vi "MGCC_EnergyMgmt_EMS_HTB_test.vi"() -> ()   [LabVIEW 2016]
uses:
  <vilib>/imath/engines/lvmath2/RunTimeEngine/NodeEndStatement/NIMS_NodeEndStatement_Output.vi
  <instcachedir>/0/NIMS_NodeEndStatement_Output_53EC0D466D134D7ABD903AC30B43404B.lvgen/NIMS_NodeEndStatement_Output_53EC0D466D134D7ABD903AC30B43404B_005.vi
  <instcachedir>/0/NIMS_NodeEndStatement_Output_53EC0D466D134D7ABD903AC30B43404B.lvgen/NIMS_NodeEndStatement_Output_53EC0D466D134D7ABD903AC30B43404B_001.vi
  <vilib>/imath/engines/lvmath2/RunTimeEngine/ErrorHandling/NIMS_Finalize Error.vi
  <vilib>/imath/engines/lvmath2/RunTimeEngine/BuiltInFunctions/is_nan/NIMS_is_nan.vi
  <instcachedir>/0/NIMS_is_nan_BCCD798162CC49E3A8E57072444F6EB6.lvgen/NIMS_is_nan_BCCD798162CC49E3A8E57072444F6EB6_003.vi
  <vilib>/imath/engines/lvmath2/RunTimeEngine/BuiltInFunctions/sum/NIMS_sum(GV).vi
  <instcachedir>/0/NIMS_sum(GV)_67F5EC36BC034E54A6BEC5B0673C00E5.lvgen/NIMS_sum(GV)_67F5EC36BC034E54A6BEC5B0673C00E5_000.vi
  <vilib>/imath/engines/lvmath2/RunTimeEngine/BuiltInFunctions/max/1 input/NIMS_max(RV).vi
  <instcachedir>/0/NIMS_max(RV)_237633DB1D604D5BA7001287DF3C7957.lvgen/NIMS_max(RV)_237633DB1D604D5BA7001287DF3C7957_002.vi
  <vilib>/imath/engines/lvmath2/RunTimeEngine/MatrixToken/NIMS_MatrixToken_RV_RV.vi
  <instcachedir>/0/NIMS_MatrixToken_RV_RV_41289AEE7DB340EFBB9CA44FA48DA89B.lvgen/NIMS_MatrixToken_RV_RV_41289AEE7DB340EFBB9CA44FA48DA89B_002.vi
  <vilib>/imath/engines/lvmath2/RunTimeEngine/MatrixToken/NIMS_MatrixToken_M_SorCV.vi
  <instcachedir>/0/NIMS_MatrixToken_M_SorCV_D3266533510A4291A747E91CF193467A.lvgen/NIMS_MatrixToken_M_SorCV_D3266533510A4291A747E91CF193467A_000.vi
  <vilib>/imath/engines/lvmath2/RunTimeEngine/ErrorHandling/NIMS_Create Error From Enums.vi
  <vilib>/imath/engines/lvmath2/RunTimeEngine/BuiltInFunctions/tril/NIMS_tril.vi
  <instcachedir>/0/NIMS_tril_6D22CCA5CB604C1FB8874D0E0A590B2C.lvgen/NIMS_tril_6D22CCA5CB604C1FB8874D0E0A590B2C_003.vi
  <vilib>/imath/engines/lvmath2/RunTimeEngine/RowToken/NIMS_RowToken_M_M.vi
  <instcachedir>/0/NIMS_RowToken_M_M_968CDE3545E74ACDAEA4B48DE01EEECA.lvgen/NIMS_RowToken_M_M_968CDE3545E74ACDAEA4B48DE01EEECA_005.vi
  <vilib>/imath/engines/lvmath2/RunTimeEngine/RowToken/NIMS_RowToken_M_CV.vi
  <instcachedir>/0/NIMS_RowToken_M_CV_FA79F1D1D17D44459F3ED8E09EE8B625.lvgen/NIMS_RowToken_M_CV_FA79F1D1D17D44459F3ED8E09EE8B625_002.vi
  <vilib>/imath/engines/lvmath2/RunTimeEngine/MatrixToken/NIMS_MatrixToken_M_M.vi
  <instcachedir>/0/NIMS_MatrixToken_M_M_DF273B0CC20F424BBF1EDA9F4E71C841.lvgen/NIMS_MatrixToken_M_M_DF273B0CC20F424BBF1EDA9F4E71C841_005.vi
  <vilib>/imath/engines/lvmath2/RunTimeEngine/ArithmeticOperatorToken/NIMS_ArithmeticOperator_minus.vi
  <instcachedir>/0/NIMS_ArithmeticOperator_minus_E3B65B1D26A44BB184AFDC5B3F458E3D.lvgen/NIMS_ArithmeticOperator_minus_E3B65B1D26A44BB184AFDC5B3F458E3D_003.vi
  <vilib>/imathl/engines/lvmath/Functions/Error Handling/Create Error.vi
  <vilib>/imath/engines/lvmath2/RunTimeEngine/BuiltInFunctions/double/NIMS_double.vi
  <instcachedir>/0/NIMS_double_34E32F64C2B04A25A042F4CA881A0A41.lvgen/NIMS_double_34E32F64C2B04A25A042F4CA881A0A41_000.vi
  <instcachedir>/0/NIMS_double_34E32F64C2B04A25A042F4CA881A0A41.lvgen/NIMS_double_34E32F64C2B04A25A042F4CA881A0A41_002.vi
  <vilib>/imath/engines/lvmath2/RunTimeEngine/BuiltInFunctions/length/NIMS_length(GV).vi
  <instcachedir>/0/NIMS_length(GV)_08A3D13377FD4E4B96F5795FBF3698FA.lvgen/NIMS_length(GV)_08A3D13377FD4E4B96F5795FBF3698FA_000.vi
  <vilib>/imath/engines/lvmath2/RunTimeEngine/BuiltInFunctions/zeros/NIMS_V=zeros(I32,I32).vi
  <vilib>/imath/engines/lvmath2/RunTimeEngine/BuiltInFunctions/ones/NIMS_V=ones(I32,I32).vi
  <vilib>/imath/engines/lvmath2/RunTimeEngine/RangeToken/NIMS_Range_R2 - Integer.vi
  <instcachedir>/0/NIMS_Range_R2 - Integer_89B873E74E6E489885E44F751DD9C6BF.lvgen/NIMS_Range_R2 - Integer_89B873E74E6E489885E44F751DD9C6BF_000.vi
  <vilib>/imath/engines/lvmath2/RunTimeEngine/CommandStatement/MC_CommandStatement_break.vi
  <vilib>/imath/engines/lvmath2/RunTimeEngine/IndexRead/NIMS V(S).vi
  <instcachedir>/0/NIMS V(S)_0488751826AF41519A22953C041130DC.lvgen/NIMS V(S)_0488751826AF41519A22953C041130DC_000.vi
  <vilib>/imath/engines/lvmath2/RunTimeEngine/BuiltInFunctions/is_inf/NIMS_is_inf.vi
  <instcachedir>/0/NIMS_is_inf_B756F33AF9174A0299BAA1DAC25DCC60.lvgen/NIMS_is_inf_B756F33AF9174A0299BAA1DAC25DCC60_002.vi
  <vilib>/imath/engines/lvmath2/RunTimeEngine/IndexReplace/NIMS V(S)=S.vi
  <instcachedir>/0/NIMS V(S)=S_57E16554CB8B4B90AAB163894F717546.lvgen/NIMS V(S)=S_57E16554CB8B4B90AAB163894F717546_003.vi
  <instcachedir>/0/NIMS_MatrixToken_M_M_DF273B0CC20F424BBF1EDA9F4E71C841.lvgen/NIMS_MatrixToken_M_M_DF273B0CC20F424BBF1EDA9F4E71C841_004.vi
  <vilib>/imath/engines/lvmath2/RunTimeEngine/BuiltInFunctions/findnz/NIMS_[3o]_findnz(GM).vi
  <instcachedir>/0/NIMS_[3o]_findnz(GM)_99A5867F30DB48758370F82C3149E97C.lvgen/NIMS_[3o]_findnz(GM)_99A5867F30DB48758370F82C3149E97C_003.vi
  <vilib>/imath/engines/lvmath2/RunTimeEngine/MatrixToken/NIMS_MatrixToken_SorCV_M.vi
  <instcachedir>/0/NIMS_MatrixToken_SorCV_M_667D6DA9EAAA4E73AD685CBB2779BCDB.lvgen/NIMS_MatrixToken_SorCV_M_667D6DA9EAAA4E73AD685CBB2779BCDB_000.vi
  <instcachedir>/0/NIMS_NodeEndStatement_Output_53EC0D466D134D7ABD903AC30B43404B.lvgen/NIMS_NodeEndStatement_Output_53EC0D466D134D7ABD903AC30B43404B_004.vi
  <instcachedir>/0/NIMS_NodeEndStatement_Output_53EC0D466D134D7ABD903AC30B43404B.lvgen/NIMS_NodeEndStatement_Output_53EC0D466D134D7ABD903AC30B43404B_010.vi
  <vilib>/imath/engines/lvmath2/RunTimeEngine/IndexRead/NIMS V(R2).vi
  <instcachedir>/0/NIMS V(R2)_C76619605A0E4E9F8B2FA9389712AC47.lvgen/NIMS V(R2)_C76619605A0E4E9F8B2FA9389712AC47_000.vi
  <instcachedir>/0/NIMS_max(RV)_237633DB1D604D5BA7001287DF3C7957.lvgen/NIMS_max(RV)_237633DB1D604D5BA7001287DF3C7957_000.vi
  <vilib>/imath/engines/lvmath2/RunTimeEngine/ArithmeticOperatorToken/NIMS_ArithmeticOperator_times.vi
  <instcachedir>/0/NIMS_ArithmeticOperator_times_953B34F74CAC448FB707D816A29CC5F0.lvgen/NIMS_ArithmeticOperator_times_953B34F74CAC448FB707D816A29CC5F0_000.vi
  liblp_solver.so
panel:
  out "Net load after":dbl[](graph)
  out "Net load b4":dbl[](graph)
  out "Battery2 Dispatch":dbl[](graph)
  out "Battery1 Dispatch":dbl[](graph)
  out "Savings":dbl
  out "return type":i32
  out "error out":errorcluster
  out "Forecast PV":dbl[](graph)
  out "Forecast Load":dbl[](graph)
  out "err_flg":i32
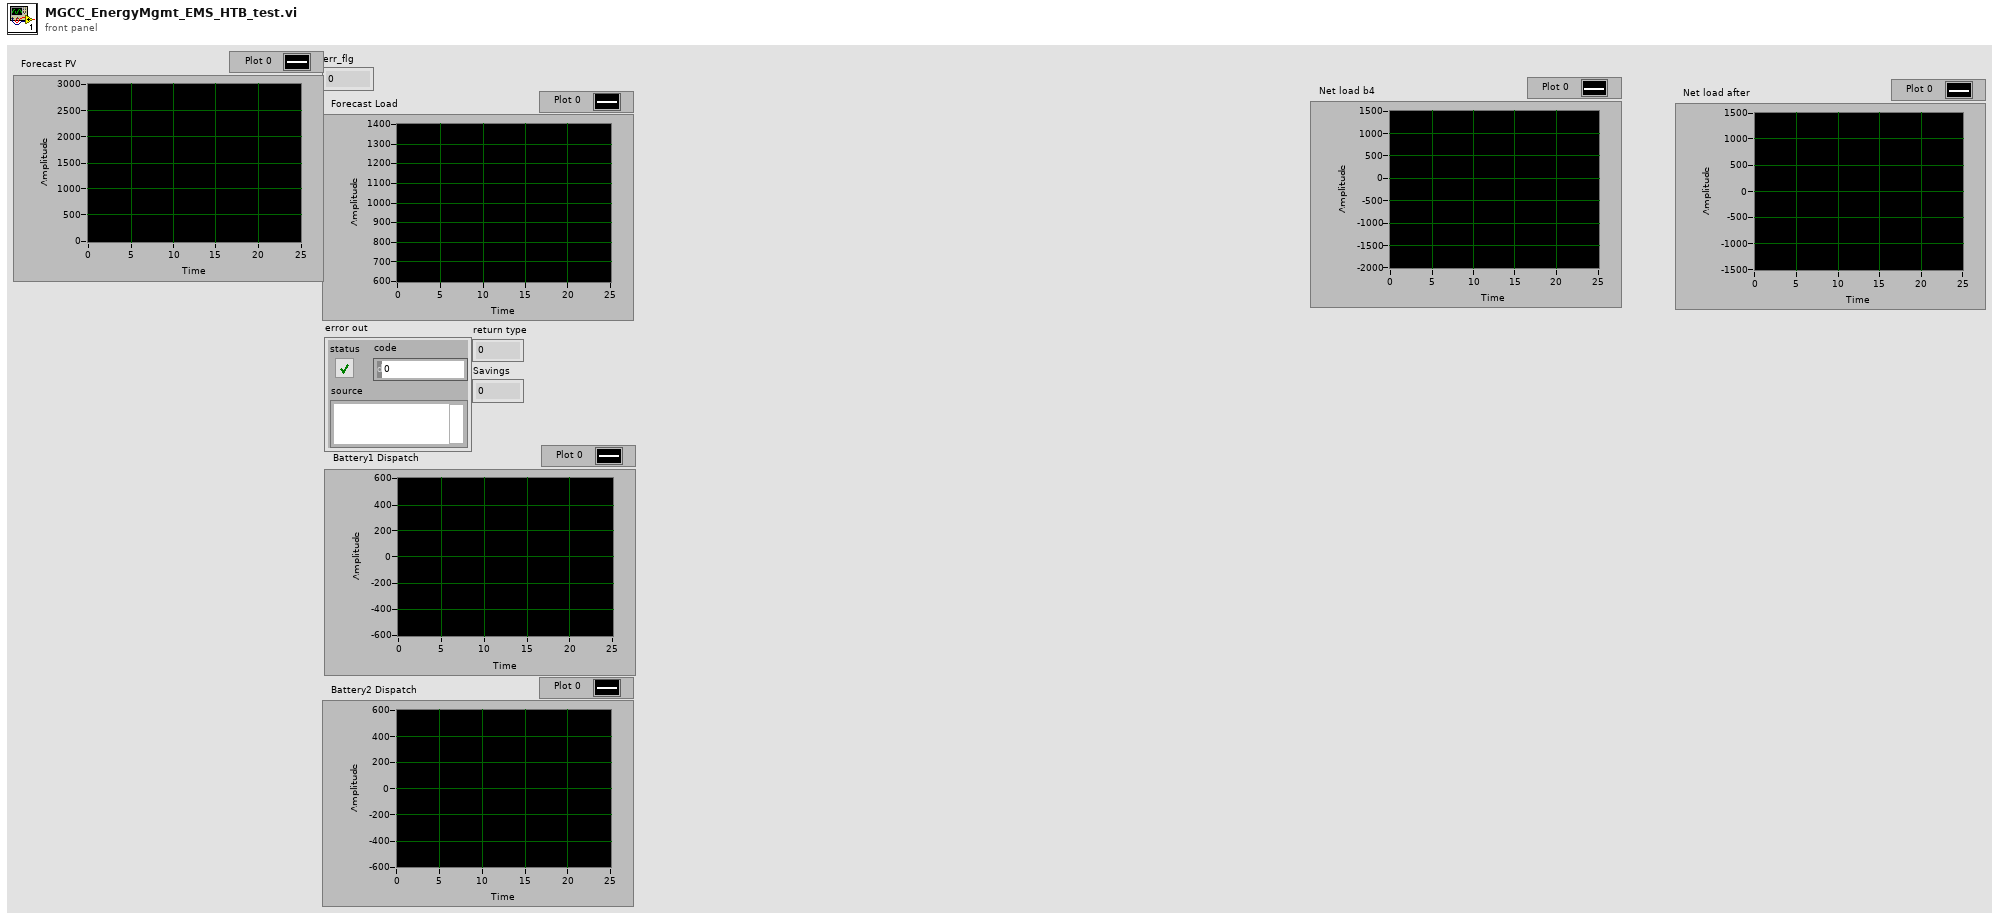
[diagram p1: front panel]
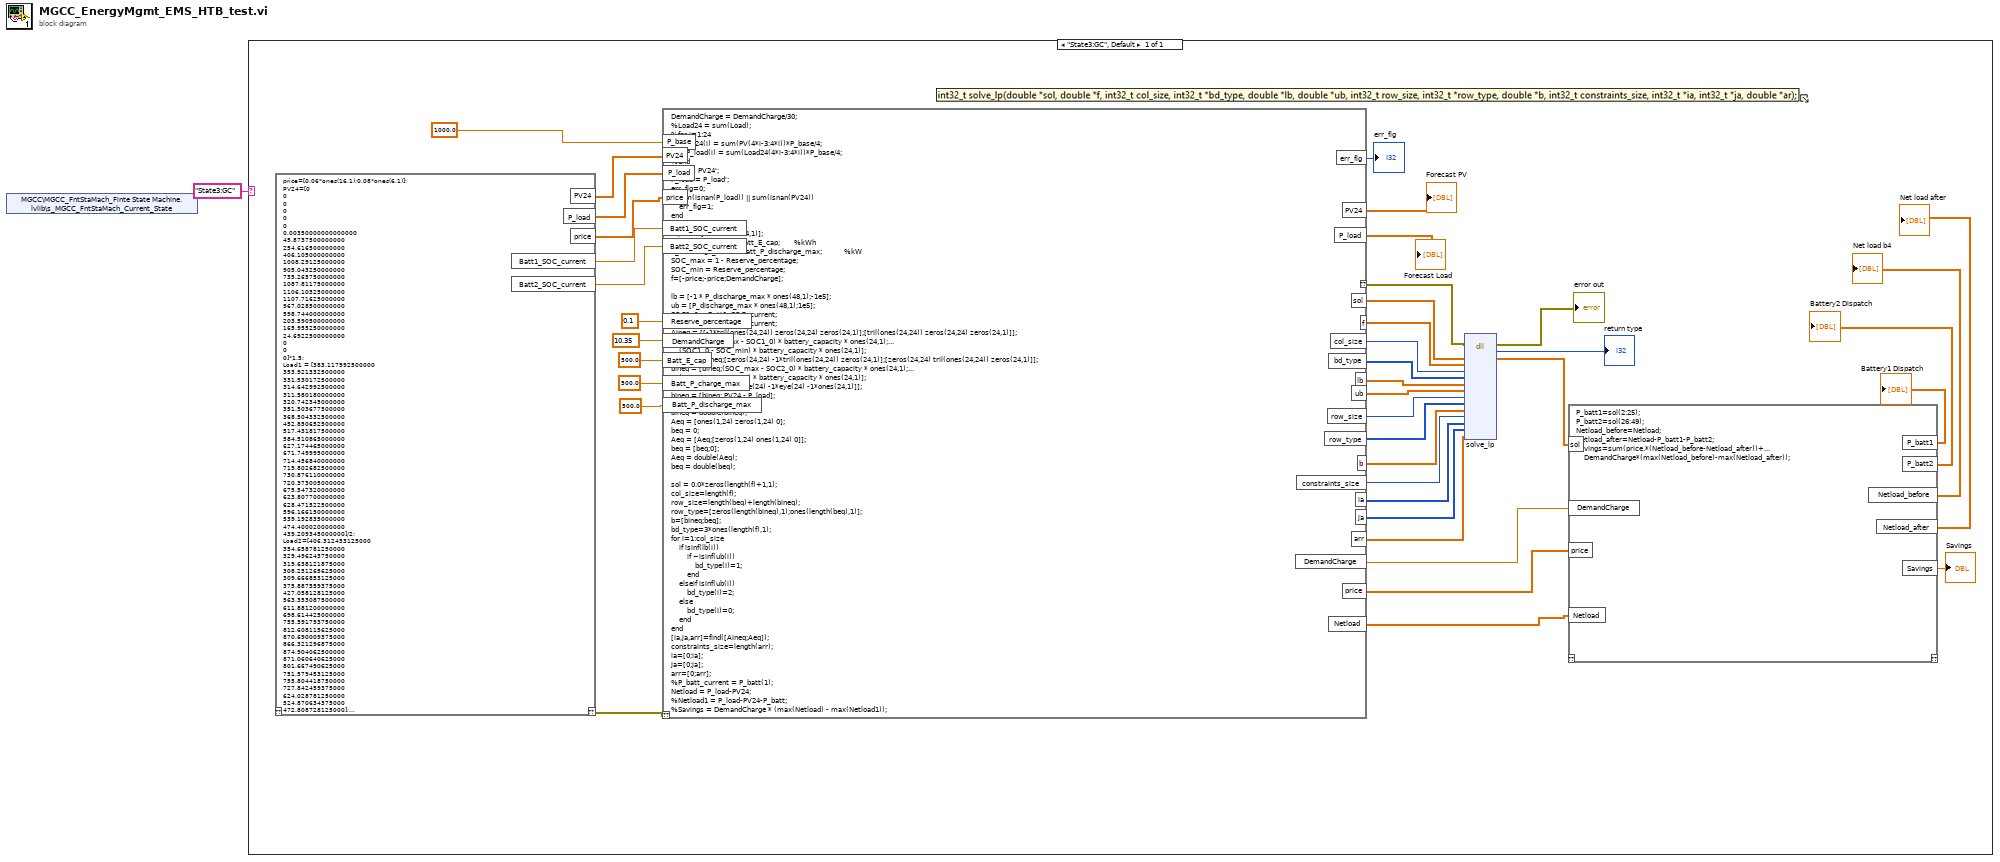
[diagram p0: block diagram]
diagram:
  n1 = shared-variable "MGCC\\MGCC_FntStaMach_Finte State Machine.lvlib\\s_MGCC_FntStaMach_Current_State"() -> ()  [unwired: 1 in, 2 out]
  n2 = case shown="\"State3:GC\", Default" "State3:GC" {
    frame "State3:GC", Default {
      n3 = mathscript code="price=[0.06*ones(16,1);0.08*ones(6,1)];\nPV24=[0\n0\n0\n0\n0\n0\n0.00350000000000000\n45.8737500000000\n254.616500000000\n406.105000000000\n1008.29125000000\n905.043250000000\n735.265750000000\n1087.81175000000\n1106.10325000000\n1107.71625000000\n967.028500000000\n598.744000000000\n203.590500000000\n165.955250000000\n24.6922500000000\n0\n0\n0]*1.5;\nLoad1 = [383.117992500000\n353.921332500000\n331.530172500000\n314.642992500000\n311.580180000000\n320.742345000000\n351.503677500000\n368.504332500000\n452.850652500000\n517.431817500000\n584.510865000000\n627.174465000000\n671.749995000000\n714.456840000000\n719.802682500000\n730.876110000000\n720.373005000000\n675.547320000000\n623.807700000000\n628.471522500000\n596.166150000000\n539.192835000000\n474.400020000000\n439.209345000000]/2;\nLoad2=[406.312453125000\n354.658781250000\n329.496243750000\n319.638121875000\n308.251265625000\n309.666853125000\n375.887559375000\n427.058128125000\n563.353087500000\n611.881200000000\n698.614425000000\n755.591793750000\n812.608115625000\n870.690009375000\n866.321296875000\n874.904062500000\n871.060640625000\n801.667490625000\n751.579453125000\n755.804418750000\n727.842459375000\n624.028781250000\n524.870634375000\n472.808728125000];\nLoad3=[998.508105000000\n988.619895000000\n934.793055000000\n865.015965000000\n883.077030000000\n933.520140000000\n906.181875000000\n844.439985000000\n914.374035000000\n1146.57106500000\n1271.49903000000\n1345.15305000000\n1430.15400000000\n1500.53301000000\n1546.58794500000\n1585.56366000000\n1534.84398000000\n1487.94795000000\n1337.79195000000\n1352.25499500000\n1247.90103000000\n1238.26491000000\n1166.81409000000\n1122.26814000000];\nLoad4=Load1*1.25;\nLoad5=Load2*1.25;\nLoad6=Load3*1.25;\nLoad7=Load1*0.5;\nP_load=Load1+Load2+Load3+Load4+Load5+Load6+Load7;\nBatt1_SOC_current=0.4;\nBatt2_SOC_current=0.6;"() -> ("??"=w30:errorcluster, "PV24"=w35:dbl[], "P_load"=w34:dbl[], "Batt1_SOC_current"=w33:dbl, "Batt2_SOC_current"=w32:dbl, "price"=w31:dbl[])  [unwired: 1 in]
      n4 = mathscript code="DemandCharge = DemandCharge/30;\n%Load24 = sum(Load);\n%for i=1:24\n%    PV24(i) = sum(PV(4*i-3:4*i))*P_base/4;\n%    P_load(i) = sum(Load24(4*i-3:4*i))*P_base/4;\n%end\nPV24 = PV24';\nP_load = P_load';\nerr_flg=0;\nif sum(isnan(P_load)) || sum(isnan(PV24))\n    err_flg=1;\nend\nerr_flg=max(err_flg);\n%price=[0.06*ones(24,1)];\nbattery_capacity = Batt_E_cap;       %kWh\nP_discharge_max = Batt_P_discharge_max;           %kW\nSOC_max = 1 - Reserve_percentage;\nSOC_min = Reserve_percentage;\nf=[-price;-price;DemandCharge];\n\nlb = [-1 * P_discharge_max * ones(48,1);-1e5];\nub = [P_discharge_max * ones(48,1);1e5];\nSOC1_0 = Batt1_SOC_current;\nSOC2_0 = Batt2_SOC_current;\nAineq = [[-1*tril(ones(24,24)) zeros(24,24) zeros(24,1)];[tril(ones(24,24)) zeros(24,24) zeros(24,1)]];\nbineq = [(SOC_max - SOC1_0) * battery_capacity * ones(24,1);...\n    (SOC1_0 - SOC_min) * battery_capacity * ones(24,1)];\nAineq = [Aineq;[zeros(24,24) -1*tril(ones(24,24)) zeros(24,1)];[zeros(24,24) tril(ones(24,24)) zeros(24,1)]];\nbineq = [bineq;(SOC_max - SOC2_0) * battery_capacity * ones(24,1);...\n    (SOC2_0 - SOC_min) * battery_capacity * ones(24,1)];\nAineq = [Aineq; [-1*eye(24) -1*eye(24) -1*ones(24,1)]];\nbineq = [bineq; PV24 - P_load];\nAineq = double(Aineq);\nbineq = double(bineq);\nAeq = [ones(1,24) zeros(1,24) 0];\nbeq = 0;\nAeq = [Aeq;[zeros(1,24) ones(1,24) 0]];\nbeq = [beq;0];\nAeq = double(Aeq);\nbeq = double(beq);\n\nsol = 0.0*zeros(length(f)+1,1);\ncol_size=length(f);\nrow_size=length(beq)+length(bineq);\nrow_type=[zeros(length(bineq),1);ones(length(beq),1)];\nb=[bineq;beq];\nbd_type=3*ones(length(f),1);\nfor i=1:col_size\n    if isinf(lb(i))\n        if ~isinf(ub(i))\n            bd_type(i)=1;\n        end\n    elseif isinf(ub(i))\n        bd_type(i)=2;\n    else\n        bd_type(i)=0;\n    end\nend\n[ia,ja,arr]=find([Aineq;Aeq]);\nconstraints_size=length(arr);\nia=[0;ia];\nja=[0;ja];\narr=[0;arr];\n%P_batt_current = P_batt(1);\nNetload = P_load-PV24;\n%Netload1 = P_load-PV24-P_batt;\n%Savings = DemandCharge * (max(Netload) - max(Netload1));"("??"=w30, "price"=w31, "Batt_E_cap"=500.0, "Batt_P_charge_max"=500.0, "Batt_P_discharge_max"=500.0, "DemandCharge"=10.35, "Reserve_percentage"=0.1, "P_base"=1000.0, "Batt1_SOC_current"=w33, "Batt2_SOC_current"=w32, "PV24"=w35, "P_load"=w34) -> ("??"=w26:errorcluster, "err_flg"=→"err_flg":i32, "PV24"=→"Forecast PV":dbl[], "P_load"=→"Forecast Load":dbl[], "sol"=w23:dbl[], "f"=w22:dbl[], "col_size"=w21:i32, "bd_type"=w20:i32[], "lb"=w19:dbl[], "ub"=w18:dbl[], "row_size"=w17:i32, "row_type"=w16:i32[], "b"=w15:dbl[], "constraints_size"=w14:i32, "ia"=w13:i32[], "ja"=w12:i32[], "arr"=w11:dbl[], "DemandCharge"=w9:dbl, "price"=w8:dbl[], "Netload"=w7:dbl[])
      n5 = dll-call lib="liblp_solver.so" fn="solve_lp"(error in=w26, "sol"=w23, "f"=w22, "col_size"=w21, "bd_type"=w20, "lb"=w19, "ub"=w18, "row_size"=w17, "row_type"=w16, "b"=w15, "constraints_size"=w14, "ia"=w13, "ja"=w12, "ar"=w11) -> (error out=→"error out":errorcluster, "return type"=→"return type":i32, "sol"=w10:dbl[])  [unwired: 14 in, 1 out]
      n6 = mathscript code="P_batt1=sol(2:25);\nP_batt2=sol(26:49);\nNetload_before=Netload;\nNetload_after=Netload-P_batt1-P_batt2;\nSavings=sum(price.*(Netload_before-Netload_after))+...\n    DemandCharge*(max(Netload_before)-max(Netload_after));"("sol"=w10, "price"=w8, "DemandCharge"=w9, "Netload"=w7) -> ("P_batt1"=→"Battery1 Dispatch":dbl[], "P_batt2"=→"Battery2 Dispatch":dbl[], "Netload_before"=→"Net load b4":dbl[], "Netload_after"=→"Net load after":dbl[], "Savings"=→"Savings":dbl)  [unwired: 1 in, 1 out]
    }
  }
